vi "MarkerStyle.vi"(10 "Marker Style":string) -> (2 "Used Marker Style":string)   [LabVIEW 2023]
uses:
  <vilib>/Utility/error.llb/whitespace.ctl
  <vilib>/Utility/error.llb/Trim Whitespace One-Sided.vi
panel:
  out "Error":bool
  out "Possible Marker Styles":string[](array[string])
  in  "Default":string="."
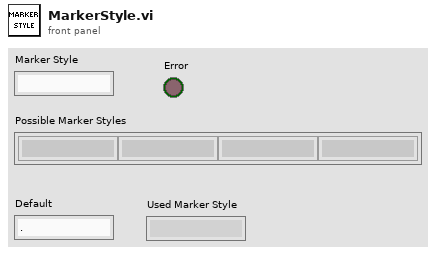
[diagram p1: front panel]
types:
  T1 = typedef "whitespace.ctl" = u16
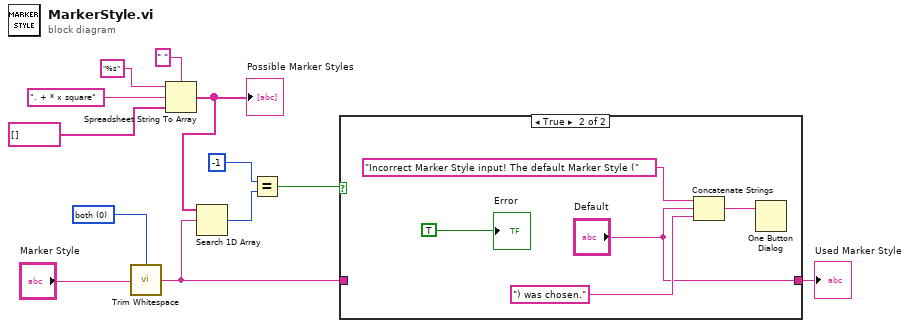
[diagram p0: block diagram]
diagram:
  w3 = T1 0 items=["both", "start of string", "end of string"] ("location (both)")
  n1 = call <vilib>:"Trim Whitespace.vi"("string"="Marker Style", "location (both)"=w3) -> ("trimmed string"=w5:string)
  n2 = Spreadsheet String To Array(delimiter (Tab)=" ", format string="%s", spreadsheet string=". + * x square", array type (2D Dbl)=string[] []) -> (array=w4:string[])
  "Possible Marker Styles" <- w4
  n3 = Search 1D Array(1D array=w4, element=w5) -> (index of element=w8:i32)  [unwired: 1 in]
  n4 = Equal?(x=-1, y=w8) -> (x = y?=w6:bool)
  n5 = case shown="True" w6 {
    tunnel: w5 -> [w13 _]
    tunnel: [w13 "Default"] -> w2
    frame False {
    }
    frame True {
      n6 = Concatenate Strings("Incorrect Marker Style input! The default Marker Style (", "Default", ") was chosen.") -> (w14:string)
      n7 = One Button Dialog(message=w14) -> ()  [unwired: 1 in, 1 out]
      "Error" <- TRUE
    }
  }
  "Used Marker Style" <- w2
